vi "NeuNet_Sub.vi"() -> ()   [LabVIEW 2015]
uses:
  <userlib>/ROS for LabVIEW Software/ROS/Code/Console/Servers/ServerSubs/TopicDef.ctl
  <userlib>/ROS for LabVIEW Software/ROS/Code/SubVIs/_ROSDirection.ctl
panel:
  out "error out":errorcluster
  in  "Stop Button":bool
  out "String":string
  in  "Definitions":T1={"Topic"="/neural_net", "Type"="std_msgs/String", "Action"=enum."Subscriber", "Update (ms)"=1, "queue size"=100}
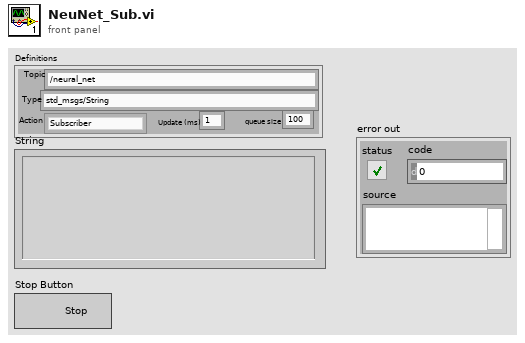
[diagram p1: front panel]
types:
  T1 = typedef "TopicDef.ctl" = cluster{"Topic":string, "Type":string, "Action":T2, "Update (ms)":u16, "queue size":u16}
  T2 = typedef "_ROSDirection.ctl" = enum16{"Node", "Publisher", "Subscriber", "ServiceClient", "ServiceProvider"}
  T3 = typedef "_ROSControl.ctl" = cluster{"topic port":u16, "Node":string, "topic":string, "type":string, "node port":u16, "error ":errorcluster, "Direction":T2, "Update (ms)":u16, "FIFO size":u16}
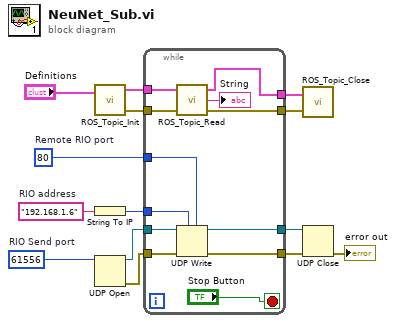
[diagram p0: block diagram]
diagram:
  w4 = u16 80  # Remote RIO port
  w8 = u16 61556  # RIO Send port
  w9 = "192.168.1.6"  # RIO address
  n1 = call <userlib>:"ROS_Topic_Init.vi"("Definitions"="Definitions") -> ("ROS out"=w11:T3, "error out"=w10:errorcluster)  [unwired: 2 in]
  n2 = String To IP(1:w9) -> (0:w5:u32)
  n3 = UDP Open(11:w8) -> (port=w7:refnum<k16>, 0:w6:errorcluster)  [unwired: 4 in, 1 out]
  n4 = while {
    tunnel: [w25] -> w14
    tunnel: [w22] -> w13
    tunnel: w11 -> [w23]
    tunnel: w10 -> [w24]
    tunnel: w7 -> [w21]
    tunnel: w6 -> [w18]
    tunnel: w5 -> [w20]
    tunnel: w4 -> [w19]
    tunnel: [w17] -> w3
    tunnel: [w16] -> w2
    stop <- "Stop Button" stop-if-true
    n5 = call <userlib>:"ROS_Topic_Read.vi"("error in (no error)"=w24, "ROS in"=w23) -> ("error out"=w22:errorcluster, "Reply"=→"String":string, "ROS out"=w25:T3)  [unwired: 1 in]
    n6 = UDP Write(address=w20, port or service name=w19, connection ID=w21, 8:w18) -> (error out=w16:errorcluster, 3:w17:refnum<k16>)  [unwired: 2 in]
  }
  n7 = call <userlib>:"ROS_Topic_Close.vi"("error in"=w13, "ROS in"=w14) -> ()  [unwired: 2 in, 1 out]
  n8 = UDP Close(connection ID=w3, 8:w2) -> (error out=→"error out":errorcluster)  [unwired: 1 out]
